vi "Mixer.MuteAudioStream.vi"(7 "value":bool) -> ()   [LabVIEW 2020]
uses:
  Typedefs/Mixer.Channel Property Data.ctl
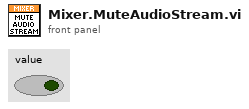
[diagram p1: front panel]
types:
  T1 = typedef "Mixer.Channel Property Data.ctl" = cluster{"channel":string, "property":string, "value":bool}
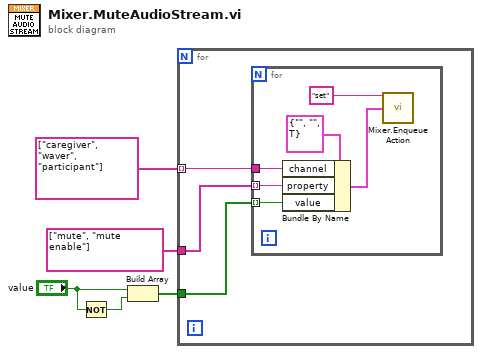
[diagram p0: block diagram]
diagram:
  n1 = Not(x="value") -> (.not. x?=w2:bool)
  n2 = Build Array("value", w2) -> (w1:bool[])
  n3 = for {
    tunnel: string[] ["caregiver", "waver", "participant"] -> [w8] mode=indexing
    tunnel: string[] ["mute", "mute enable"] -> [w7]
    tunnel: w1 -> [w6]
    n4 = for {
      tunnel: w8 -> [w11]
      tunnel: w7 -> [w10] mode=indexing
      tunnel: w6 -> [w9] mode=indexing
      n5 = Bundle By Name(cluster=T1 {"channel"="", "property"="", "value"=TRUE} ("Cluster"), "channel"=w11, "property"=w10, "value"=w9) -> (w14:T1)
      n6 = call "Mixer.Enqueue Action.vi"("action"="set", "data"=w14) -> ()  [unwired: 13 in, 1 out]
    }
  }
